vi "BWC_CollectDMDImagingCalibration.vi"() -> ()   [LabVIEW 2017]
panel:
  out "concatenated string 3":string="C:\\Users\\1TEM\\Documents\\1TEM_control\\tem_image_acquisition\\bin\\Release\\tem_image_acquisition.exe --gain 50 --exposure 1000 --blacklvl 180 --filename \"calib_SPOT_1024__768_capture.png\""
  out "standard error":string
  out "concatenated string 2":string="--gain 50 --exposure 1000 --blacklvl 180 --filename \"calib_SPOT_1024__768_capture.png\""
  out "standard output":string="Initializing camera ...\r\nSuccess!\r\nGetting sensor info ...\r\nSuccess!\r\nCamera ID: 1\r\nSensor dimensions: 1600 x 1200 (assuming bit-depth per pixel of 24)\r\nAllocating memory for images ...\r\nSuccess!\r\nSetting image memory location ...\r\nSuccess!\r\nGetting current exposure ...\r\nSuccess!\r\nCurrent exposure: 25.1076 ms\r\nGetting current frame rate ...\r\nSuccess!\r\nCurrent frame rate 39.7962\r\n\r\nSuccess!\r\nSuccess!\r\nSuccess!\r\nSetting frame rate to 0.1 fps ...\r\nSuccess!\r\nFrame rate set to 0.99985 fps ...\r\n\r\nGetting valid exposure range ...\r\nSuccess!\r\nMin: 0.0201 ms\r\nMax: 999.98 ms\r\nInc: 0.170122 ms\r\nSetting new exposure to: 1000 ms ...\r\nSuccess!\r\nCurrent exposure now 999.98 ms\r\n\r\nGetting current gain ...\r\nCurrent gain setting is: 0\r\nSuccess!\r\nSetting gain to 50 ...\r\nSuccess!\r\nGetting current gain ...\r\nCurrent gain setting is: 50\r\n\r\nSuccess!\r\nGetting current blacklevel ...\r\nSuccess!\r\nCurrent blacklevel: 132\r\nSetting blacklevel to 180...\r\nSuccess!\r\nGetting current blacklevel ...\r\nSuccess!\r\nCurrent blacklevel: 180\r\n\r\nFreezing video ...\r\nSuccess!\r\n\r\nFreezing video ...\r\nSuccess!\r\n\r\nSaving image ...\r\n\r\nSaving image to calib_SPOT_1024__768_capture.png ...\r\nSuccess!\r\n\r\nShutting down camera ...\r\n"
  in  "ImagePath":path=path "\\\\LEO1272\\Caplins/Calibrations"
  in  "opts":string="--gain 50 --exposure 1000 --blacklvl 180"
  in  "program name":string="tem_image_acquisition.exe"
  in  "program path":path=path "C:/Users/1TEM/Documents/1TEM_control/tem_image_acquisition/bin/Release"
  # "Steps:\n1. Set up microscope for illumination of DMD\n2. Push masks to DMD\n3. Collect/save image\n\n4. Ideally, do analysis... but maybe matlab/octave is easier..."
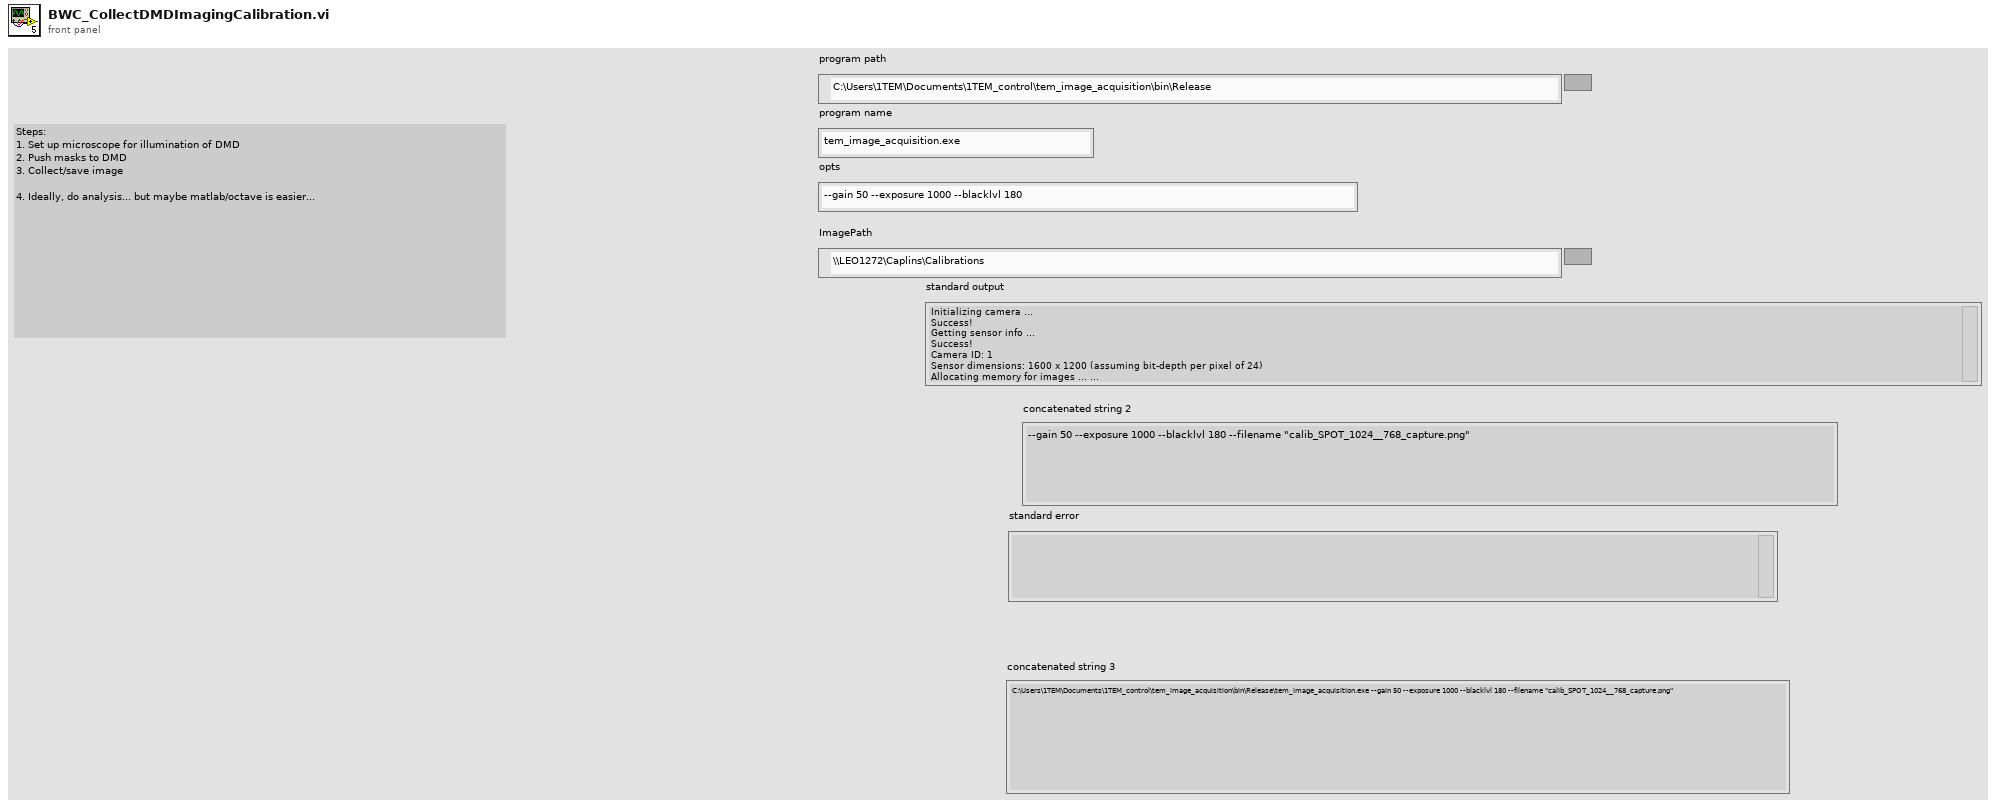
[diagram p1: front panel]
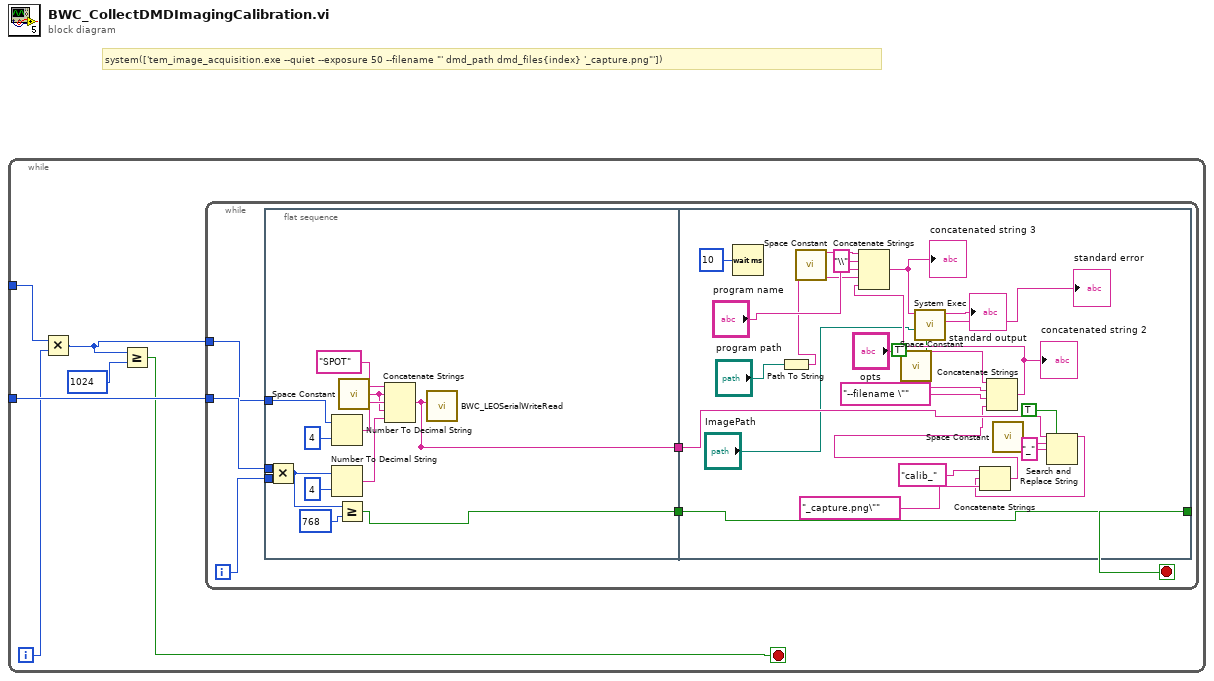
[diagram p0: block diagram]
diagram:
  # "system(['tem_image_acquisition.exe --quiet --exposure 50 --filename \"' dmd_path dmd_files{index} '_capture.png\"'])"
  n1 = while {
    tunnel: [w8] -> w1
    tunnel: [w7] -> w2
    i -> [w6]
    stop <- w4 stop-if-true
    n2 = Multiply(x=w7, y=w6) -> (x*y=w3:i32)
    n3 = Greater Or Equal?(x=w3, y=1024) -> (x >= y?=w4:bool)
    n4 = while {
      tunnel: w3 -> [w11]
      tunnel: w8 -> [w14]
      i -> [w13]
      stop <- w12 stop-if-true
      n5 = flat-sequence {
        tunnel: w14 -> [w30]
        tunnel: w13 -> [w29]
        tunnel: [w27] -> w10
        tunnel: w11 -> [w24]
        tunnel: [w15] -> w9
        tunnel: [w52] -> w12
        tunnel: w10 -> [w52]
        tunnel: w9 -> [w45]
        frame #0 {
          n6 = Multiply(x=w30, y=w29) -> (x*y=w23:i32)
          n7 = Number To Decimal String(number=w24, width (-)=i16 4) -> (decimal integer string=w22:string)
          n8 = Number To Decimal String(number=w23, width (-)=i16 4) -> (decimal integer string=w20:string)
          n9 = Greater Or Equal?(x=w23, y=768) -> (x >= y?=w27:bool)
          n10 = call <vilib>:"Space Constant.vi"() -> ("String"=w19:string)
          n11 = Concatenate Strings("SPOT" ("Command To Write"), w19, w22, w19, w20) -> (w15:string)
          n12 = call "BWC_LEOSerialWriteRead.vi"("Command To Write"=w15) -> ("error out"=w16:errorcluster, "Completion Response"=w17:string, "Acknowledge Response"=w18:string)  [unwired: 6 in, 1 out]
        }
        frame #1 {
          n13 = Wait (ms)(milliseconds to wait=u32 10) -> ()  [unwired: 1 out]
          n14 = Path To String(path="program path") -> (string=w33:string)
          n15 = call <vilib>:"Space Constant.vi"() -> ("String"=w38:string)
          n16 = call <vilib>:"Space Constant.vi"() -> ("String"=w47:string)
          n17 = call <vilib>:"Space Constant.vi"() -> ("String"=w43:string)
          n18 = Search and Replace String(replace all?=TRUE ("replace all? (F)"), input string=w45, search string=w43, replace string="_" ("replace string (\"\")")) -> (result string=w41:string)  [unwired: 4 in, 3 out]
          n19 = Concatenate Strings("calib_", w41, "_capture.png\"" ("string")) -> (w35:string)
          n20 = Concatenate Strings("opts", w47, "--filename \"", w35) -> (w39:string)
          "concatenated string 2" <- w39
          n21 = Concatenate Strings(w33, "\\" ("string"), "program name", w38, w39) -> (w37:string)
          "concatenated string 3" <- w37
          n22 = call <vilib>:"System Exec.vi"("run minimized? (F)"=TRUE, "working directory"="ImagePath", "command line"=w37) -> ("standard error"=→"standard error":string, "standard output"=→"standard output":string)  [unwired: 5 in, 2 out]
        }
      }
    }
  }
